vi "evenodd.vi"() -> ()   [LabVIEW 2019]
panel:
  out "info":string
  in  "Numeric":dbl
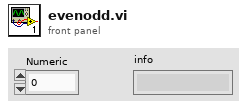
[diagram p1: front panel]
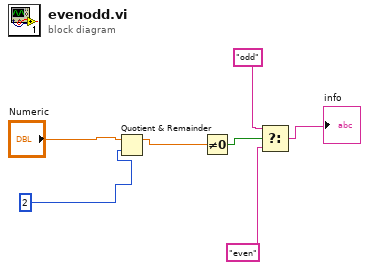
[diagram p0: block diagram]
diagram:
  n1 = Quotient & Remainder(x="Numeric", y=2) -> (x-y*floor(x/y)=w5:dbl)  [unwired: 1 out]
  n2 = Not Equal To 0?(x=w5) -> (x != 0?=w2:bool)
  n3 = Select(t="odd", s=w2, f="even") -> (s? t:f=→"info":string)
